vi "Class.vi"(7 "Config":refnum<class "TAF Proj Config.lvclass">, 8 "error in":errorcluster, 11 "Library Ref":refnum<vi>) -> (0 "error out":errorcluster, 3 "Class out":refnum<class "Class.lvclass">)   [LabVIEW 2021, in "TAF Proj Document Type.lvlib" / "Project Parser.lvlib"]
uses:
  <vilib>/Wovalab/AntiDoc/Document Type/Add-ons/LabVIEW TAF Project/Project Parser/Project Parser.lvlib
  <vilib>/Wovalab/AntiDoc/Document Type/Add-ons/LabVIEW TAF Project/Class/Class.lvclass
  C:/Program Files (x86)/National Instruments/LabVIEW 2021/vi.lib/Wovalab/AntiDoc/Document Type/Add-ons/LabVIEW TAF Project/Lib/Lib.lvclass
  <vilib>/Wovalab/AntiDoc/Document Type/Add-ons/LabVIEW TAF Project/TAF Proj Config/TAF Proj Config.lvclass
  <vilib>/Wovalab/AntiDoc/Document Type/Add-ons/LabVIEW TAF Project/Class/Class.lvclass/Class.ctl
  <vilib>/Wovalab/AntiDoc/Document Type/Add-ons/LabVIEW TAF Project/Class/Write Is Interface.vi
  <vilib>/Wovalab/AntiDoc/Document Type/Add-ons/LabVIEW TAF Project/Class/Write Uml.vi
  <vilib>/Wovalab/AntiDoc/classy-diagram-viewer/classyDiagramViewer.lvlib
panel:
  out "Private Data Control":refnum<vi>
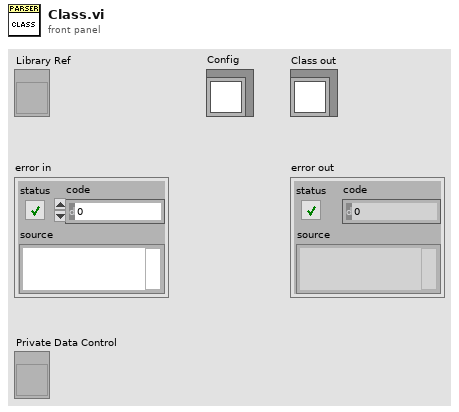
[diagram p1: front panel]
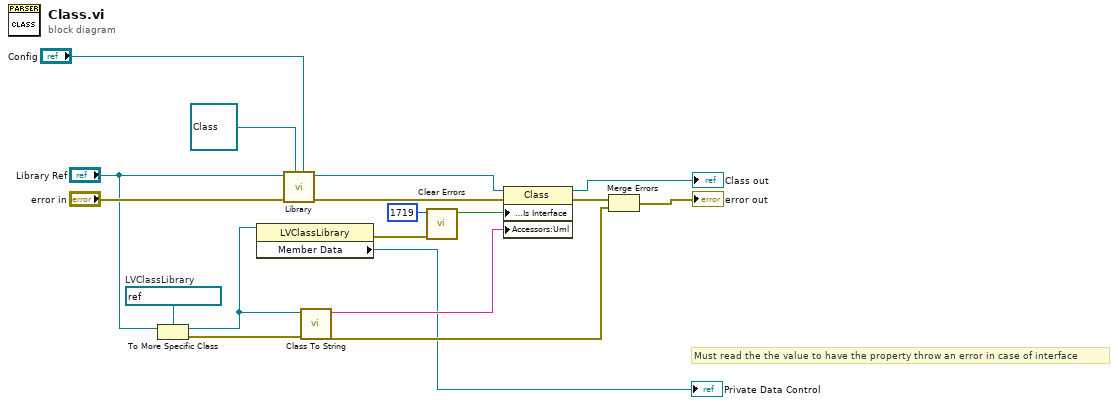
[diagram p0: block diagram]
diagram:
  w11 = refnum<vi> refnum  # LVClassLibrary
  # "Must read the the value to have the property throw an error in case of interface"
  n1 = To More Specific Class(target class=w11, reference="Library Ref") -> (specific class reference=w4:refnum<vi>, error out=w18:errorcluster)  [unwired: 1 in]
  n2 = property class="LVClassLibrary"(reference=w4) -> (error out=w12:errorcluster, "Member Data"=→"Private Data Control":refnum<vi>)  [unwired: 1 in, 1 out]
  n3 = call <vilib>:"Library.vi"("Config"="Config", "Lib Type"=refnum<class "Class.lvclass"> refnum ("Antidoc:Class.lvclass"), "error in"="error in", "Library Ref"="Library Ref") -> ("error out"=w16:errorcluster, "Lib out"=w9:refnum<class "Class.lvclass">)  [unwired: 6 in]
  n4 = call <vilib>:"Class To String.vi"("error in (no error)"=w18, "class reference"=w4) -> ("error out"=w13:errorcluster, "plantUML string"=w5:string)  [unwired: 8 in]
  n5 = call <vilib>:"Clear Errors.vi"("error in (no error)"=w12, "specific error code to clear (0: all)"=1719 ("error code (no error:0)")) -> ("specific error cleared?"=w2:bool)  [unwired: 4 in, 1 out]
  n6 = property class="Class"(reference=w9, error in=w16, "Accessors:Is Interface"=w2, "Accessors:Uml"=w5) -> (reference out=→"Class out":refnum<class "Class.lvclass">, error out=w15:errorcluster)
  n7 = Merge Errors(w15, w13) -> (→"error out":errorcluster)
